vi "Set Out.vi"(8 "error in":errorcluster, 11 "FPGA-DIO in":refnum<class "FPGA_DIO.lvclass">) -> (0 "error out":errorcluster, 3 "FPGA-DIO out":refnum<class "FPGA_DIO.lvclass">)   [LabVIEW 2019, in "FPGA_DIO.lvlib" / "FPGA_DIO.lvclass"]
uses:
  Library/FPGA_DIO.lvclass
  C:/Users/Public/Documents/Development/builds/Instruments/DIG_IO.lvlibp/Library/DIG_IO.lvclass
  Library/FPGA_DIO.lvclass/FPGA_DIO.ctl
  builds/Instruments/DIG_IO.lvlibp/Accessors/Read Digital.vi
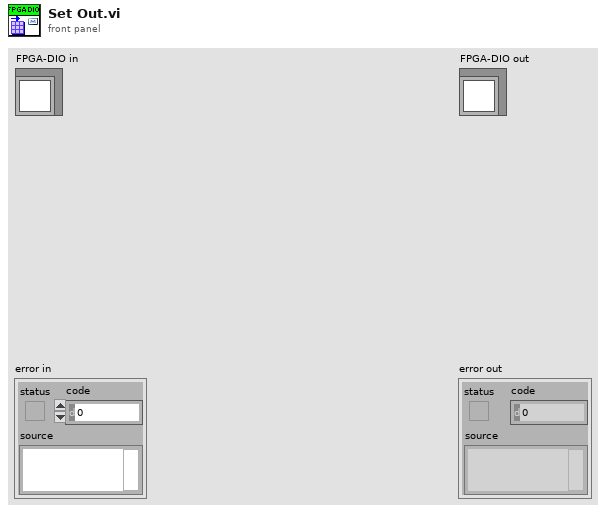
[diagram p1: front panel]
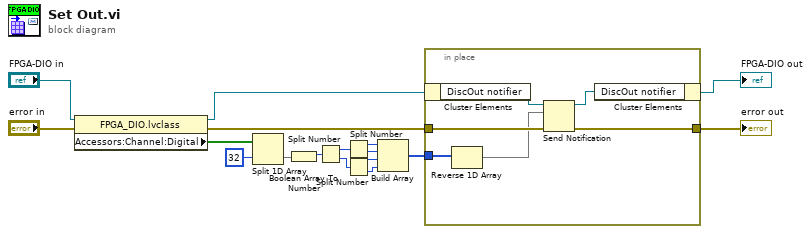
[diagram p0: block diagram]
diagram:
  n1 = property class="FPGA_DIO.lvclass"(reference="FPGA-DIO in", error in="error in") -> (reference out=w15:refnum<class "FPGA_DIO.lvclass">, error out=w13:errorcluster, "Accessors:Channel:Digital"=w11:bool[])
  n2 = Split 1D Array(array=w11, index=32) -> (second subarray=w9:bool[])  [unwired: 1 out]
  n3 = Boolean Array To Number(Boolean array=w9) -> (number=w8:u32)
  n4 = Split Number(x=w8) -> (hi(x)=w7:u16, lo(x)=w6:u16)
  n5 = Split Number(x=w7) -> (hi(x)=w5:u8, lo(x)=w4:u8)
  n6 = Split Number(x=w6) -> (hi(x)=w3:u8, lo(x)=w2:u8)
  n7 = Build Array(w5, w4, w3, w2) -> (w1:u8[])
  n8 = in-place {
    in-place-border: w13 -> [w21]
    in-place-border: [w20] -> w12
    in-place-border: w1 -> [w19]
    n9 = in-place-cluster #1(w15) -> ("DiscOut notifier"=w23:refnum<notifier>)
    n10 = Reverse 1D Array(array=w19) -> (reversed array=w18:u8[])
    n11 = Send Notification(notification=w18, notifier=w23, error in (no error)=w21) -> (notifier out=w22:refnum<notifier>, error out=w20:errorcluster)
    n12 = in-place-cluster #1("DiscOut notifier"=w22) -> (→"FPGA-DIO out":refnum<class "FPGA_DIO.lvclass">)
  }
  "error out" <- w12
